vi "ReturnValues.vi"(6 "error in":errorcluster, 9 "Diagram in":refnum<class "Diagram.lvclass">) -> (0 "error out":errorcluster, 3 "Diagram out":refnum<class "Diagram.lvclass">, 4 "inputs":string[](array[string]), 5 "return":string)   [LabVIEW 2014, in "Diagram.lvclass"]
uses:
  Diagram.lvclass
  Python/Parsing/ListTypesTD.ctl
  Terminal/Terminal.lvclass
  Python/Parsing/Python Functions.lvlib
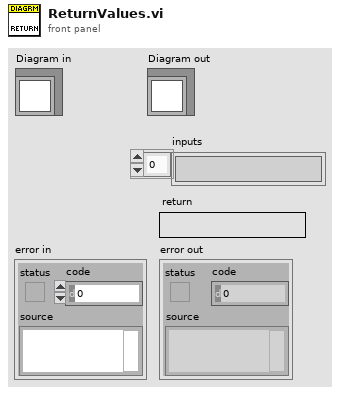
[diagram p1: front panel]
types:
  T1 = typedef "Python Functions.lvlib/ListTypesTD.ctl" = enum16{"list", "tuple", "parameter list", "output list"}
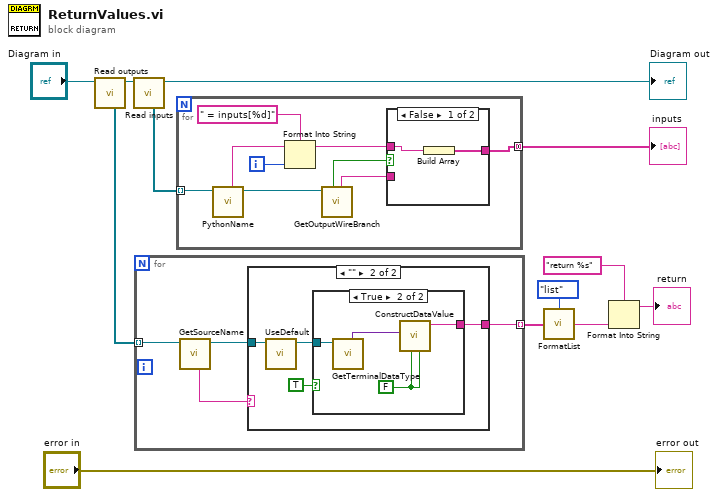
[diagram p0: block diagram]
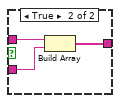
[diagram p4: hidden frame]
diagram:
  n1 = call-dynamic "Read outputs.vi"("Diagram in"="Diagram in") -> ("Diagram out"=w3:refnum<class "Diagram.lvclass">, "outputs"=w4:refnum<class "Terminal.lvclass">[])  [unwired: 7 in]
  n2 = call-dynamic "Read inputs.vi"("Diagram in"=w3) -> ("Diagram out"=→"Diagram out":refnum<class "Diagram.lvclass">, "inputs"=w5:refnum<class "Terminal.lvclass">[])  [unwired: 7 in]
  n3 = for {
    tunnel: [w16] -> w11 mode=indexing
    tunnel: w4 -> [w15] mode=indexing
    n4 = call "GetSourceName.vi"("Terminal in"=w15) -> ("Terminal out"=w14:refnum<class "Terminal.lvclass">, "source"=w13:string)  [unwired: 6 in, 1 out]
    n5 = case shown="\"\"" w13 {
      selector: w13 -> [w17 _]
      tunnel: [w17 w19] -> w16
      tunnel: w14 -> [_ w21]
      frame Default {
      }
      frame "" {
        n6 = call "UseDefault.vi"("Terminal in"=w21) -> ("Terminal out"=w20:refnum<class "Terminal.lvclass">)  [unwired: 6 in, 2 out]
        n7 = case shown="True" TRUE {
          tunnel: w20 -> [_ w25]
          tunnel: [_ w24] -> w19
          frame False {
          }
          frame True {
            w22 = FALSE ("label")
            n8 = call "GetTerminalDataType.vi"("Terminal in"=w25) -> ("Data Type"=w23:variant)  [unwired: 6 in, 2 out]
            n9 = call "ConstructDataValue.vi"("label"=w22, "value"=w22, "Value"=w23) -> ("value"=w24:string)  [unwired: 6 in]
          }
        }
      }
    }
  }
  n10 = for {
    tunnel: [w26] -> w12 mode=concatenating
    tunnel: w5 -> [w31] mode=indexing
    i -> [w33]
    n11 = call-dynamic "PythonName.vi"("Terminal in"=w31) -> ("Terminal out"=w30:refnum<class "Terminal.lvclass">, "name"=w34:string)  [unwired: 7 in, 2 out]
    n12 = Format Into String(format string=" = inputs[%d]", initial string=w34, w33) -> (resulting string=w27:string)  [unwired: 1 in, 1 out]
    n13 = call-dynamic "GetOutputWireBranch.vi"("Terminal in"=w30) -> ("branches"=w28:string, "branched"=w29:bool)  [unwired: 5 in, 2 out]
    n14 = case shown="False" w29 {
      tunnel: w28 -> [_ w38]
      tunnel: w27 -> [w36 w39]
      tunnel: [w35 w37] -> w26
      frame False {
        n15 = Build Array(w36) -> (w35:string[])
      }
      frame True {
        n16 = Build Array(w39, w38) -> (w37:string[])
      }
    }
  }
  "inputs" <- w12
  n17 = call "FormatList.vi"("values"=w11, "type"=ListTypesTD."list") -> ("python object"=w9:string)
  n18 = Format Into String(format string="return %s", w9) -> (resulting string=→"return":string)  [unwired: 2 in, 1 out]
  "error out" <- "error in"
